vi "Apply Lookup Table.vi"(0 "RFmx Instrument Handle In":refnum<k21> caption="Instrument Handle In", 1 "Selector String":string, 5 "SG instrument handle":refnum<k15>, 7 "Lookup Table Configuration":T1={"Threshold Enabled"=1, "Threshold Type"=0, "Threshold Level (dB)"=-20.0, "Lookup Table Step Size (dB)"=0.1, "Lookup Table Correction Type"=0, " Lookup Table Type"=0} {"Lookup Table Type" items=["Log", "Linear"]; "Lookup Table Correction Type" items=["Magnitude and Phase", "Magnitude Only", "Phase Only"]; "Threshold Level (dB)" format="%.2g"; "Threshold Type" items=["Relative", "Absolute"]; "Threshold Enabled" items=["False", "True"]}, 9 "Common Configuration":T2={"Measurement Interval (s)"=0.0001, "Sample Rate Mode"=1, "Sample Rate (Hz)"=120000000.0, "Signal Type"=0, "Pre DPD CFR Enabled"=0, "Apply DPD CFR Enabled"=0, "DUT Average Input Power (dBm)"=-15.0} {"DUT Average Input Power (dBm)" format="%.2f"; "Apply DPD CFR Enabled" items=["False", "True"]; "Pre DPD CFR Enabled" items=["False", "True"]; "Signal Type" items=["Modulated", "Tones"]; "Sample Rate (Hz)" format="%.2p"; "Sample Rate Mode" items=["User", "Reference Waveform"]; "Measurement Interval (s)" format="%#.2p"}, 11 "error in (no error)":errorcluster, 12 "Waveform":T4={"Waveform Name"="Wfm", "Waveform"={"x0"=0.0, "dx"=0.0, "y"=[]}, "Signal Bandwidth (Hz)"=0.0, "PAPR (dB)"=0.0, "Burst Length (s)"=0.0, "Sample Rate"=0.0, "Burst Start Locations"=[], "Burst Stop Locations"=[], "Idle Duration Present?"=FALSE, "Runtime Scaling"=0.0} {"Runtime Scaling" format="%#_6p"; "Sample Rate" format="%#_6p"; "Burst Length (s)" format="%#_6p"; "PAPR (dB)" format="%.2f"; "Signal Bandwidth (Hz)" format="%#_6p"; "Waveform"."y" format="%.2f"; "Waveform"."dx" format="%^.2e"; "Waveform"."x0" format="%^.2e"}) -> (4 "RFmx Instrument Handle Out":refnum<k21> caption="Instrument Handle Out", 6 "SG instrument handle out":refnum<k15>, 8 "Lookup Table Results":T3={"Post Dpd Waveform"={"x0"=0.0, "dx"=0.0, "y"=[]}, "Post Dpd Papr (dB)"=-1.0, "Power Offset (dB)"=-1.0, "Input Powers(dBm)"=[], "Complex Gains(dB)"=[]} {"Power Offset (dB)" format="%.2f"; "Post Dpd Papr (dB)" format="%.2f"; "Post Dpd Waveform"."y" format="%.2f"; "Post Dpd Waveform"."dx" format="%^.2e"; "Post Dpd Waveform"."x0" format="%^.2e"}, 15 "error out":errorcluster)   [LabVIEW 2016, in "RFmxDPD.lvlib"]
uses:
  RFmxDPD.lvlib
  SG/Typedefs/Waveform.ctl
  Typedefs/Lookup Table  Results.ctl
  Typedefs/Common Configuration.ctl
  Typedefs/Lookup Table Configuration.ctl
  <vilib>/RFmx/SpecAn/mx/RFmxSpecAn.llb/RFmxSpecAn DPD Fetch Lookup Table.vi
  SG/SG.lvlib
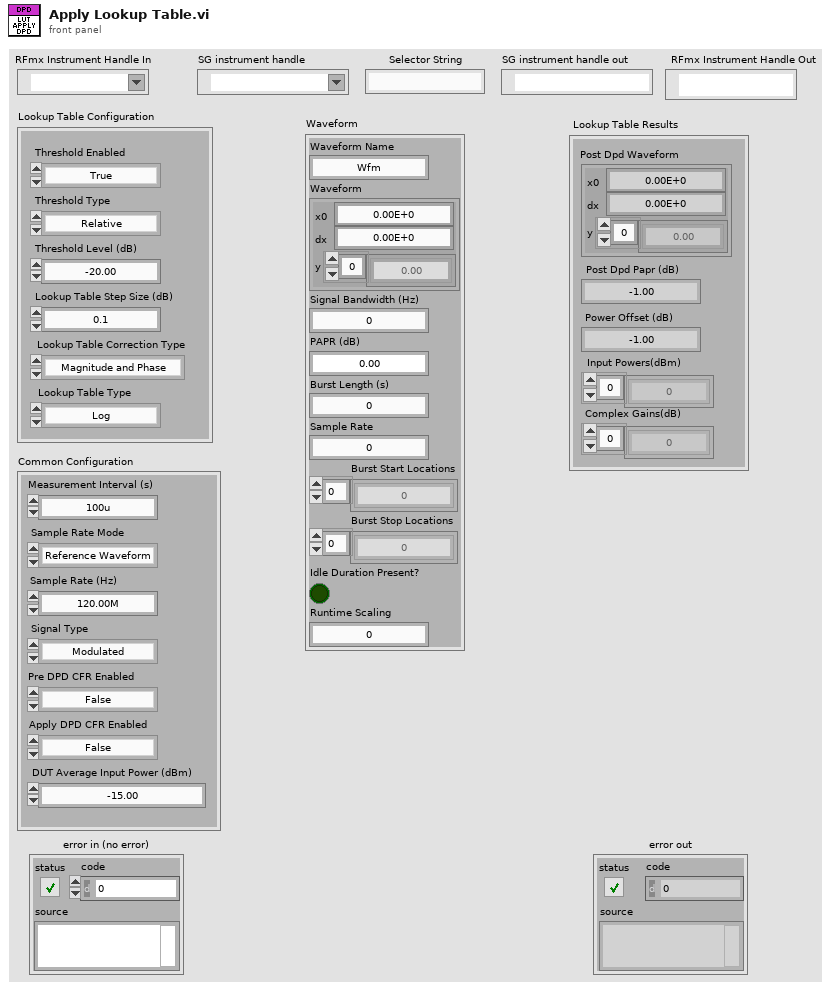
[diagram p1: front panel]
types:
  T1 = typedef "RFmxDPD.lvlib/Lookup Table Configuration.ctl" = cluster{"Threshold Enabled":i32, "Threshold Type":i32, "Threshold Level (dB)":dbl, "Lookup Table Step Size (dB)":dbl, "Lookup Table Correction Type":i32, " Lookup Table Type":i32}
  T2 = typedef "RFmxDPD.lvlib/Common Configuration.ctl" = cluster{"Measurement Interval (s)":dbl, "Sample Rate Mode":i32, "Sample Rate (Hz)":dbl, "Signal Type":i32, "Pre DPD CFR Enabled":i32, "Apply DPD CFR Enabled":i32, "DUT Average Input Power (dBm)":dbl}
  T3 = typedef "RFmxDPD.lvlib/Lookup Table  Results.ctl" = cluster{"Post Dpd Waveform":cluster{"x0":dbl, "dx":dbl, "y":csg[]}, "Post Dpd Papr (dB)":dbl, "Power Offset (dB)":dbl, "Input Powers(dBm)":sgl[], "Complex Gains(dB)":csg[]}
  T4 = typedef "SG.lvlib/Waveform.ctl" = cluster{"Waveform Name":string, "Waveform":cluster{"x0":dbl, "dx":dbl, "y":csg[]}, "Signal Bandwidth (Hz)":dbl, "PAPR (dB)":dbl, "Burst Length (s)":dbl, "Sample Rate":dbl, "Burst Start Locations":i32[], "Burst Stop Locations":i32[], "Idle Duration Present?":bool, "Runtime Scaling":dbl}
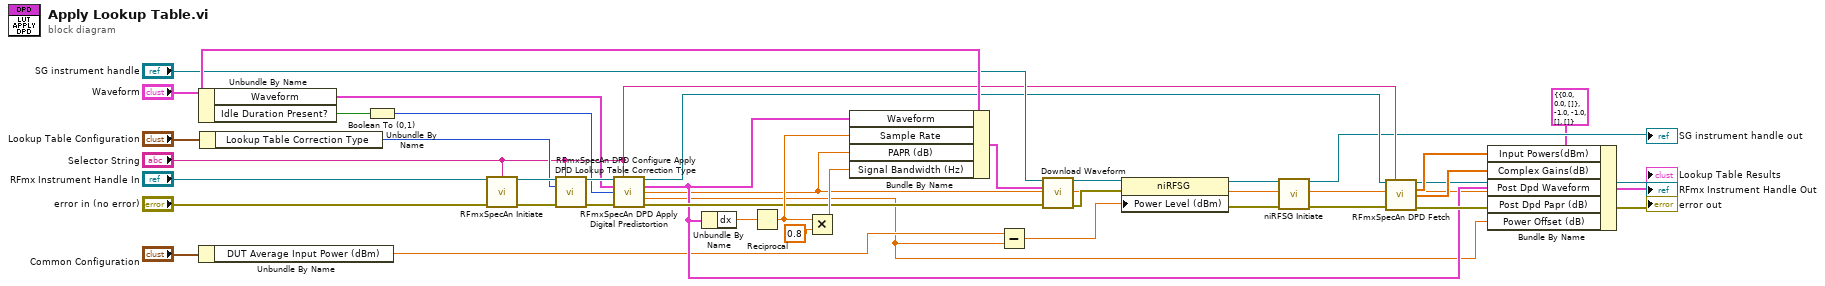
[diagram p0: block diagram]
diagram:
  n1 = Unbundle By Name("Waveform") -> ("Waveform"=w32:cluster{"x0":dbl, "dx":dbl, "y":csg[]}, "Idle Duration Present?"=w31:bool)
  n2 = Unbundle By Name("Common Configuration") -> ("DUT Average Input Power (dBm)"=w4:dbl)
  n3 = Unbundle By Name("Lookup Table Configuration") -> ("Lookup Table Correction Type"=w33:i32)
  n4 = Boolean To (0,1)(Boolean=w31) -> (0, 1=w30:i16)
  n5 = call <vilib>:"RFmxSpecAn Initiate.vi"("Instrument Handle In"="RFmx Instrument Handle In", "Result Name"="Selector String", "error in (no error)"="error in (no error)") -> ("Instrument Handle Out"=w38:refnum<k21>, "error out"=w37:errorcluster)  [unwired: 10 in, 1 out]
  n6 = call <vilib>:"RFmxSpecAn DPD Configure Apply DPD Lookup Table Correction Type.vi"("Instrument Handle In"=w38, "Selector String"="Selector String", "LUT Correction Type"=w33, "error in (no error)"=w37) -> ("Instrument Handle Out"=w36:refnum<k21>, "error out"=w35:errorcluster)  [unwired: 10 in]
  n7 = call <vilib>:"RFmxSpecAn DPD Apply Digital Predistortion.vi"("Instrument Handle In"=w36, "Selector String"="Selector String", "Waveform In"=w32, "Idle Duration Present"=w30, "error in (no error)"=w35) -> ("Instrument Handle Out"=w17:refnum<k21>, "Waveform Out"=w12:cluster{"x0":dbl, "dx":dbl, "y":csg[]}, "PAPR (dB)"=w1:dbl, "Power Offset (dB)"=w2:dbl, "error out"=w22:errorcluster)  [unwired: 6 in]
  n8 = Unbundle By Name(w12) -> ("dx"=w28:dbl)
  n9 = Reciprocal(x=w28) -> (1/x=w27:dbl)
  n10 = Multiply(x=w27, y=0.8) -> (x*y=w25:dbl)
  n11 = Bundle By Name(cluster="Waveform", "Waveform"=w12, "Sample Rate"=w27, "PAPR (dB)"=w1, "Signal Bandwidth (Hz)"=w25) -> (w23:T4)
  n12 = Subtract(x=w4, y=w2) -> (x-y=w3:dbl)
  n13 = call "Download Waveform.vi"("RFSG handle"="SG instrument handle", "Waveform In"=w23, "error in (no error)"=w22) -> ("RFSG handle out"=w21:refnum<k15>, "error out"=w20:errorcluster)  [unwired: 11 in]
  n14 = property class="niRFSG"(reference=w21, error in=w20, "Power Level (dBm)"=w3) -> (reference out=w19:refnum<k15>, error out=w18:errorcluster)
  n15 = call <instrlib>:"niRFSG Initiate.vi"("instrument handle"=w19, "error in"=w18) -> ("instrument handle out"=→"SG instrument handle out":refnum<k15>, "error out"=w16:errorcluster)  [unwired: 12 in]
  n16 = call-poly <vilib>:"RFmxSpecAn DPD Fetch.vi"("Instrument Handle In"=w17, "Selector String"="Selector String", "error in (no error)"=w16) -> ("Instrument Handle Out"=→"RFmx Instrument Handle Out":refnum<k21>, "Input Powers"=w14:sgl[], "Complex Gains"=w13:csg[], "error out"=→"error out":errorcluster)  [unwired: 9 in]
  n17 = Bundle By Name(cluster=T3 {"Post Dpd Waveform"={"x0"=0.0, "dx"=0.0, "y"=[]}, "Post Dpd Papr (dB)"=-1.0, "Power Offset (dB)"=-1.0, "Input Powers(dBm)"=[], "Complex Gains(dB)"=[]} ("Lookup Table Results"), "Input Powers(dBm)"=w14, "Complex Gains(dB)"=w13, "Post Dpd Waveform"=w12, "Post Dpd Papr (dB)"=w1, "Power Offset (dB)"=w2) -> (→"Lookup Table Results":T3)
